vi "GetGXMLCfgRes.vi"(8 "error in (no error)":errorcluster, 11 "Resistance in":refnum<class "Resistance.lvclass">) -> (0 "error out":errorcluster, 2 "ResChanCfg":T1, 3 "Resistance out":refnum<class "Resistance.lvclass">)   [LabVIEW 2012, in "Measurement Channels.lvlib" / "Resistance.lvclass"]
uses:
  Resistance.lvclass
  ResProps_TD.ctl
  Resistance.lvclass/Resistance.ctl
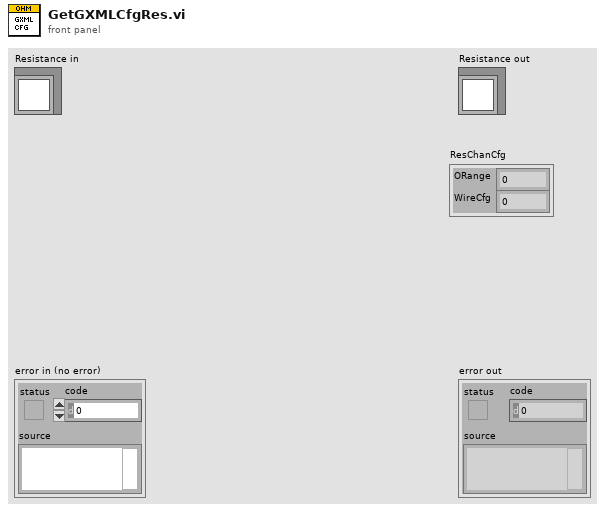
[diagram p1: front panel]
types:
  T1 = typedef "Measurement Channels.lvlib/Resistance.lvclass/ResProps_TD.ctl" = cluster{"ORange":u16, "WireCfg":u16}
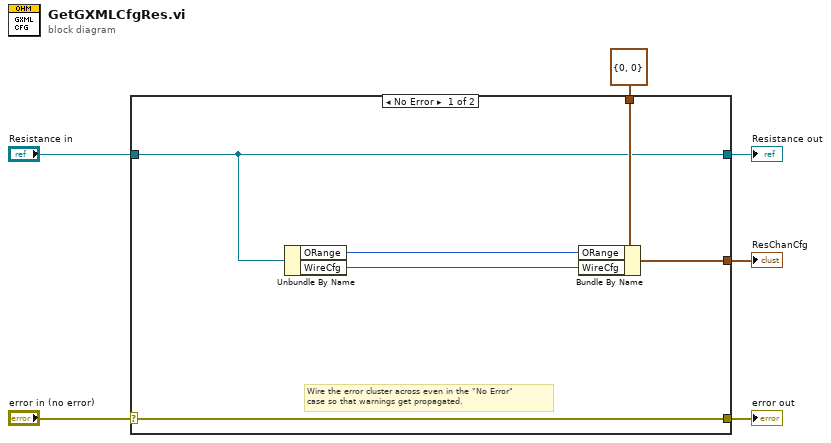
[diagram p0: block diagram]
diagram:
  n1 = case shown="No Error" "error in (no error)" {
    selector: "error in (no error)" -> [w12 w15]
    tunnel: [w12 w15] -> w5
    tunnel: [w9 w14] -> w3
    tunnel: "Resistance in" -> [w9 w14]
    tunnel: [w10 w13] -> w2
    tunnel: T1 {"ORange"=0, "WireCfg"=0} ("ResChanCfg") -> [w11 w13]
    frame No Error {
      # "Wire the error cluster across even in the \"No Error\"\ncase so that warnings get propagated."
      n2 = Unbundle By Name(w9) -> ("ORange"=w8:u16, "WireCfg"=w7:u16)
      n3 = Bundle By Name(cluster=w11, "ORange"=w8, "WireCfg"=w7) -> (w10:T1)
    }
    frame Error {
    }
  }
  "error out" <- w5
  "Resistance out" <- w3
  "ResChanCfg" <- w2
